vi "Stop Core.vi"(10 "final error code":i32, 11 "Actor_Log in":refnum<class "Actor_Log.lvclass">) -> (3 "Actor_Log out":refnum<class "Actor_Log.lvclass">)   [LabVIEW 2020, in "Library Core.lvlib" / "Actor_Log.lvlib" / "Actor_Log.lvclass"]
doc: "(<B>Filename</B>: Actor Framework.lvlib:Actor.lvclass:Stop Core.vi)\n\nDefines what the actor does before it stops. Use the <B>final error code</B> input to determine whether the actor shut down in response to an error.\n\nBy default, this method does nothing. A descendant class may override it to define behavior, such as shutting down any processes the actor initiated in its override of the Actor Core method."
uses:
  Actor_Log.lvclass
  Actor_Log.lvclass/Actor_Log.ctl
  <vilib>/ActorFramework/Actor/Actor.lvclass
  Commun VI/Library Commun.lvlib
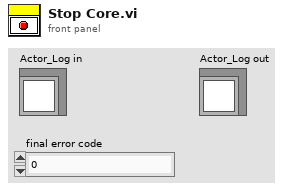
[diagram p1: front panel]
types:
  T1 = enum16{"Init", "Add Actor", "Delete Actor", "Get Actor Queue", "Get Log Actor Queue", "List all actors"}
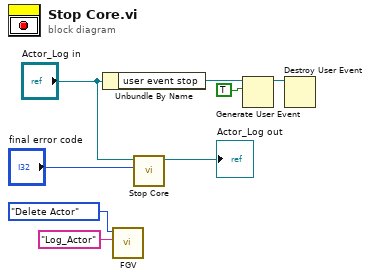
[diagram p0: block diagram]
diagram:
  n1 = Unbundle By Name("Actor_Log in") -> ("user event stop"=w5:refnum<user-event>)
  n2 = call "FGV.vi"("Actor name"="Log_Actor", "Action"=T1."Delete Actor") -> ()  [unwired: 7 in, 3 out]
  n3 = call-parent "Stop Core.vi"("final error code"="final error code", "Actor in"="Actor_Log in") -> ("Actor out"=→"Actor_Log out":refnum<class "Actor_Log.lvclass">)  [unwired: 9 in]
  n4 = Generate User Event(user event=w5, event data cluster=TRUE ("event data")) -> (user event out=w3:refnum<user-event>)  [unwired: 2 in, 1 out]
  n5 = Destroy User Event(user event=w3) -> ()  [unwired: 1 in, 1 out]
